vi "ProdaNG.WabcoPart.New.vi"(8 "error in (no error)":errorcluster, 11 "dbHandleIn":i32) -> (0 "error out":errorcluster, 3 "dbHandle":i32)   [LabVIEW 2016]
doc: "This function returns a product structure for a product, which is identified by a part and a serial number.\nImportant information: The field 'individual' was taken over from the field 'allgemein' of the legacy data directly. Because of this most products have the value 0 further on and only a few the value 1. \nParameter:\nhandle is an Integer, which is returned by the function Login() at the creation of a new connection.\nwabcoPartId is the Id of the part.\nserialNumber is the serial number of the product for the part above.\nproduct is a pointer on a product structure, which is filled if the returncode is 0. The structure must be defined in the calling program.\n\nReturncodes:\n0 No error\n< 0 ORACLE Error code\n6 (ERROR_INVALID_HANDLE) in case of an invalid handle\n1403 Record does not exist"
uses:
  Controls/ProdaNG.WabcoPart.ctl
  Controls/ProdaNG.WabcoPartSize.ctl
  prodllNG.dll
panel:
  out "WabcoPart out":T1
  in  "WabcoPart":T1
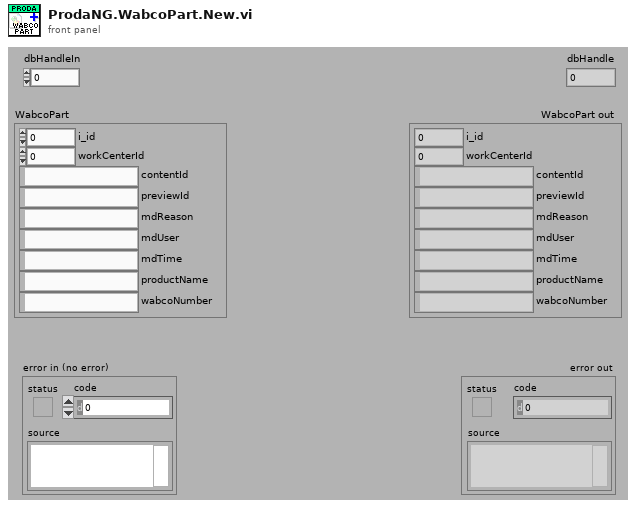
[diagram p1: front panel]
types:
  T1 = typedef "ProdaNG.WabcoPart.ctl" = cluster{"i_id":i32, "workCenterId":i32, "contentId":string, "previewId":string, "mdReason":string, "mdUser":string, "mdTime":string, "productName":string, "wabcoNumber":string}
  T2 = typedef "ProdaNG.WabcoPartSize.ctl" = cluster{"i_id":i32, "workCenterId":i32, "contentId":i32, "previewId":i32, "mdReason":i32, "mdUser":i32, "mdTime":i32, "productName":i32, "wabcoNumber":i32}
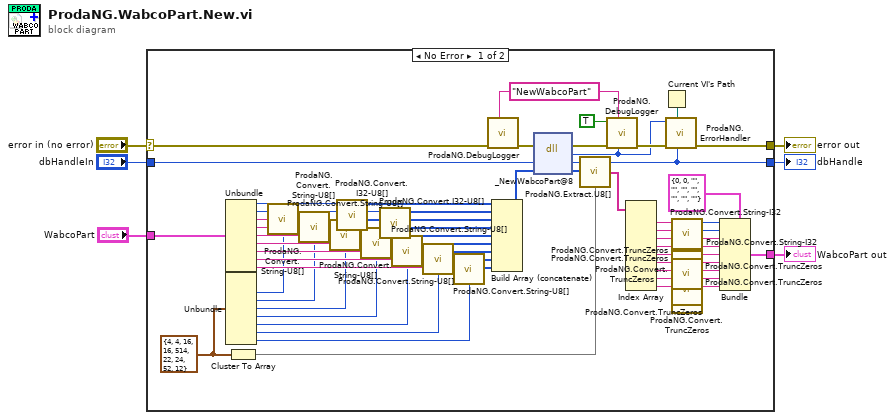
[diagram p0: block diagram]
diagram:
  n1 = case shown="No Error" "error in (no error)" {
    selector: "error in (no error)" -> [w63 w70]
    tunnel: [w68 w70] -> w5
    tunnel: "dbHandleIn" -> [w65 w69]
    tunnel: [w66 w69] -> w3
    tunnel: [w57 _] -> w2
    tunnel: "WabcoPart" -> [w21 _]
    frame No Error {
      w22 = T2 {"i_id"=4, "workCenterId"=4, "contentId"=16, "previewId"=16, "mdReason"=514, "mdUser"=22, "mdTime"=24, "productName"=52, "wabcoNumber"=12} ("WabcoPart")
      w59 = "NewWabcoPart" ("cmd")
      n2 = Unbundle(w21) -> ("i_id"=w32:i32, "workCenterId"=w33:i32, "contentId"=w17:string, "previewId"=w16:string, "mdReason"=w30:string, "mdUser"=w26:string, "mdTime"=w28:string, "productName"=w25:string, "wabcoNumber"=w18:string)
      n3 = Unbundle(w22) -> ("contentId"=w7:i32, "previewId"=w8:i32, "mdReason"=w9:i32, "mdUser"=w10:i32, "mdTime"=w11:i32, "productName"=w19:i32, "wabcoNumber"=w12:i32)  [unwired: 2 out]
      n4 = Cluster To Array(cluster=w22) -> (array=w35:i32[])
      n5 = call "ProdaNG.Convert.String-U8[].vi"("Input String"=w17, "Size"=w7) -> ("Output"=w15:u8[])
      n6 = call "ProdaNG.Convert.String-U8[].vi"("Input String"=w16, "Size"=w8) -> ("Output"=w14:u8[])
      n7 = call "ProdaNG.Convert.String-U8[].vi"("Input String"=w30, "Size"=w9) -> ("Output"=w29:u8[])
      n8 = call "ProdaNG.Convert.I32-U8[].vi"("32bit integer"=w32) -> ("unsigned byte array"=w31:u8[])  [unwired: 10 in]
      n9 = call "ProdaNG.Convert.String-U8[].vi"("Input String"=w26, "Size"=w10) -> ("Output"=w23:u8[])
      n10 = call "ProdaNG.Convert.I32-U8[].vi"("32bit integer"=w33) -> ("unsigned byte array"=w34:u8[])  [unwired: 10 in]
      n11 = call "ProdaNG.Convert.String-U8[].vi"("Input String"=w28, "Size"=w11) -> ("Output"=w27:u8[])
      n12 = call "ProdaNG.Convert.String-U8[].vi"("Input String"=w25, "Size"=w19) -> ("Output"=w24:u8[])
      n13 = call "ProdaNG.Convert.String-U8[].vi"("Input String"=w18, "Size"=w12) -> ("Output"=w13:u8[])
      n14 = call "ProdaNG.DebugLogger.vi"("cmd"=w59, "error in (no error)"=w63) -> ("error out"=w62:errorcluster)  [unwired: 9 in]
      n15 = Build Array (concatenate)(w31, w34, w15, w14, w29, w23, w27, w24, w13) -> (w20:u8[])
      n16 = dll-call lib="D:/Maszup/WABCO/SVN/LineTraceSystem/SOFTWARE/sources/Database/ProdaNG/prodllNG.dll" fn="_NewWabcoPart@8" ("ProDLL wrapper.dll:ProDLL_wrapper_GetWabcoParts_GetData")(error in=w62, "dbHandle"=w65, "wabcoPartsPtr"=w20) -> (error out=w61:errorcluster, "return type"=w58:i32, "dbHandle"=w66:i32, "wabcoPartsPtr"=w36:u8[])  [unwired: 2 in, 1 out]
      n17 = call "ProdaNG.Extract.U8[].vi"("unsigned byte array"=w36, "Sizes"=w35) -> ("Elements"=w48:string[])
      n18 = call "ProdaNG.DebugLogger.vi"("return type"=w58, "cmd"=w59, "error in (no error)"=w61, "done? (F)"=TRUE) -> ("error out"=w60:errorcluster)  [unwired: 7 in]
      n19 = Index Array(array=w48) -> (element #1=w50:string, element #2=w49:string, element #3=w41:string, element #4=w42:string, element #5=w54:string, element #6=w56:string, element #7=w47:string, element #8=w46:string, element #9=w37:string)  [unwired: 9 in]
      n20 = Current VI's Path() -> (path=w67:path)
      n21 = call "ProdaNG.ErrorHandler.vi"("dbHandleIn"=w66, "Path"=w67, "error in"=w60, "output_parameter"=w58) -> ("error out"=w68:errorcluster)  [unwired: 7 in]
      n22 = call "ProdaNG.Convert.String-I32.vi"("unsigned byte string"=w50) -> ("32bit integer"=w52:i32)  [unwired: 10 in]
      n23 = call "ProdaNG.Convert.String-I32.vi"("unsigned byte string"=w49) -> ("32bit integer"=w51:i32)  [unwired: 10 in]
      n24 = call "ProdaNG.Convert.TruncZeros.vi"("string with \\0s"=w41) -> ("LV string"=w40:string)  [unwired: 10 in]
      n25 = call "ProdaNG.Convert.TruncZeros.vi"("string with \\0s"=w42) -> ("LV string"=w39:string)  [unwired: 10 in]
      n26 = call "ProdaNG.Convert.TruncZeros.vi"("string with \\0s"=w54) -> ("LV string"=w53:string)  [unwired: 10 in]
      n27 = call "ProdaNG.Convert.TruncZeros.vi"("string with \\0s"=w56) -> ("LV string"=w55:string)  [unwired: 10 in]
      n28 = call "ProdaNG.Convert.TruncZeros.vi"("string with \\0s"=w47) -> ("LV string"=w45:string)  [unwired: 10 in]
      n29 = call "ProdaNG.Convert.TruncZeros.vi"("string with \\0s"=w46) -> ("LV string"=w44:string)  [unwired: 10 in]
      n30 = call "ProdaNG.Convert.TruncZeros.vi"("string with \\0s"=w37) -> ("LV string"=w38:string)  [unwired: 10 in]
      n31 = Bundle(cluster=T1 {"i_id"=0, "workCenterId"=0, "contentId"="", "previewId"="", "mdReason"="", "mdUser"="", "mdTime"="", "productName"="", "wabcoNumber"=""} ("WabcoPart"), "i_id"=w52, "workCenterId"=w51, "contentId"=w40, "previewId"=w39, "mdReason"=w53, "mdUser"=w55, "mdTime"=w45, "productName"=w44, "wabcoNumber"=w38) -> (w57:T1)
    }
    frame Error {
    }
  }
  "error out" <- w5
  "dbHandle" <- w3
  "WabcoPart out" <- w2
